vi "Get Cooler Status.vi"(8 "error in (no error)":errorcluster, 11 "CCDCamera in":refnum<class "Sim_Ixon_Ultra.lvclass">) -> (0 "error out":errorcluster, 3 "CCDCamera out":refnum<class "Sim_Ixon_Ultra.lvclass">)   [LabVIEW 2018, in "Sim_Ixon_Ultra.lvclass"]
doc: "Get the cooler status.\n\nThis function returns the current temperature and the temperature status. These possible values of the temperature status are stabilized, not stabilzed, or not reached."
uses:
  Sim_Ixon_Ultra.lvclass
  Sim_Ixon_Ultra.lvclass/Sim_Ixon_Ultra.ctl
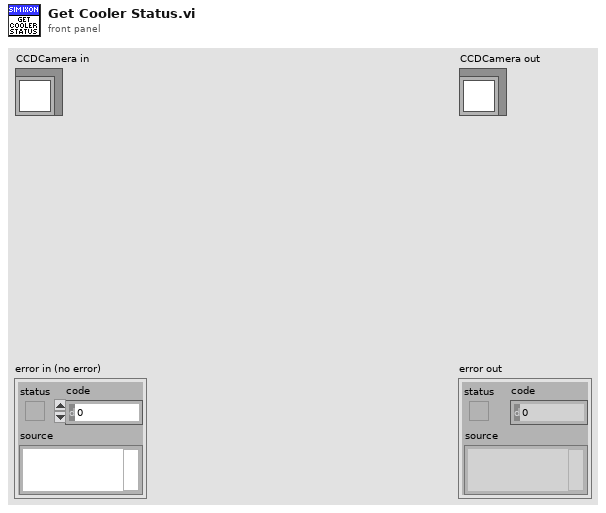
[diagram p1: front panel]
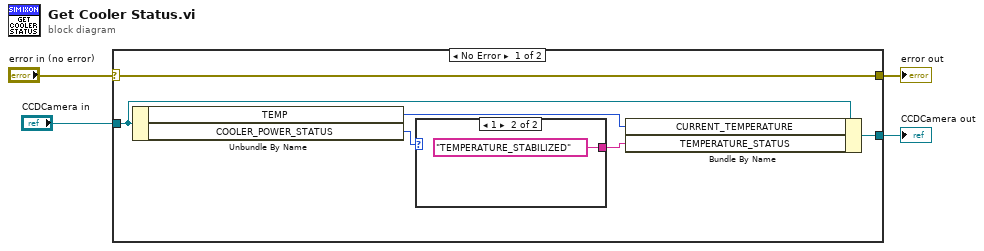
[diagram p0: block diagram]
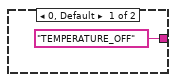
[diagram p2: hidden frame]
diagram:
  n1 = case shown="No Error" "error in (no error)" {
    selector: "error in (no error)" -> [w10 w14]
    tunnel: [w10 w14] -> w3
    tunnel: [w5 w13] -> w1
    tunnel: "CCDCamera in" -> [w6 w13]
    frame No Error {
      n2 = Unbundle By Name(w6) -> ("TEMP"=w9:i32, "COOLER_POWER_STATUS"=w7:u16)
      n3 = case shown="1" w7 {
        tunnel: ["TEMPERATURE_OFF" ("TEMPERATURE_STATUS") "TEMPERATURE_STABILIZED" ("TEMPERATURE_STATUS")] -> w8
        frame 0, Default {
        }
        frame 1 {
        }
      }
      n4 = Bundle By Name(cluster=w6, "CURRENT_TEMPERATURE"=w9, "TEMPERATURE_STATUS"=w8) -> (w5:refnum<class "Sim_Ixon_Ultra.lvclass">)
    }
    frame Error {
    }
  }
  "error out" <- w3
  "CCDCamera out" <- w1
